vi "_getTempValueOfAllPortsTemp_EEPROM_VNA_wmg.vi"(0 "AA or AB?":bool=TRUE, 5 "portNum":i32, 7 "ref_W&R_ports":refnum<vi>[](array[refnum]), 9 "AA or AB inf":i32[](array[numeric]), 11 "info_write":string[][](array[string])) -> (4 "temp port0":string[][](array[string]), 6 "temp port1":string[][](array[string]), 10 "temp port2":string[][](array[string]), 14 "temp port4":string[][](array[string]), 15 "temp port3":string[][](array[string]))   [LabVIEW 2011]
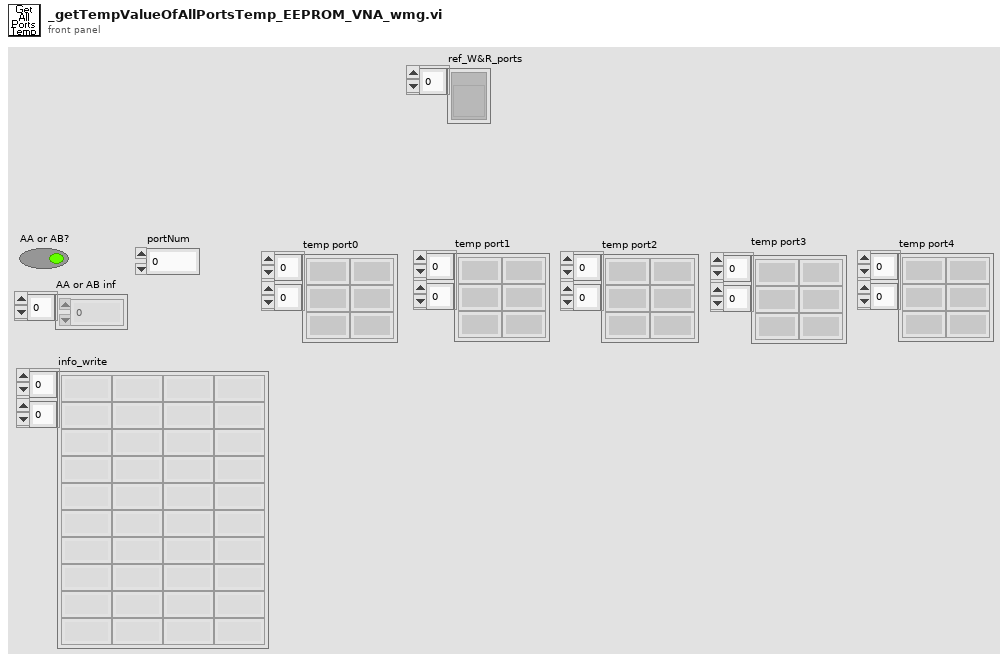
[diagram p1: front panel]
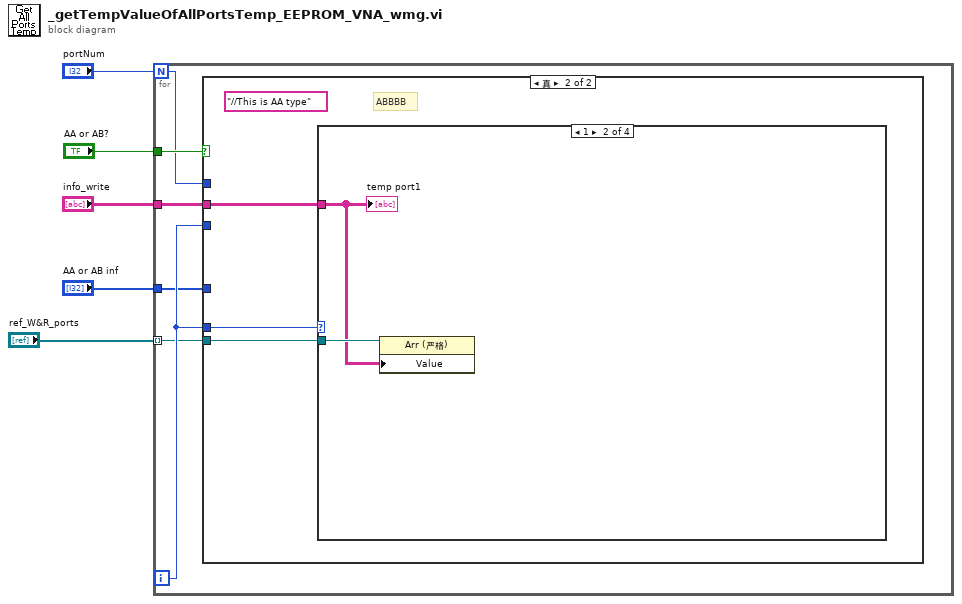
[diagram p0: block diagram]
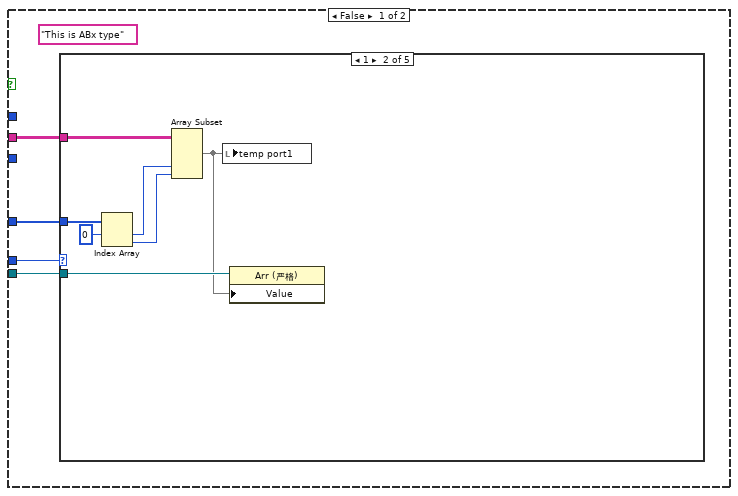
[diagram p2: hidden frame]
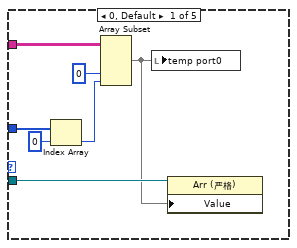
[diagram p3: hidden frame]
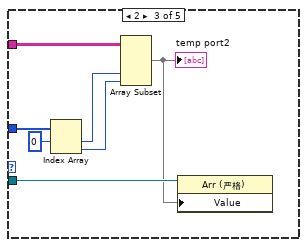
[diagram p4: hidden frame]
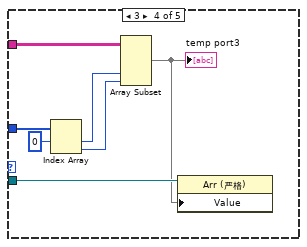
[diagram p5: hidden frame]
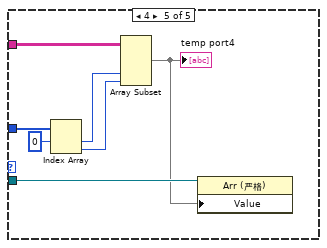
[diagram p6: hidden frame]
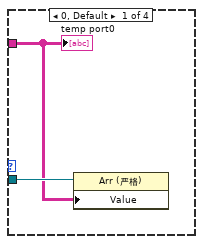
[diagram p7: hidden frame]
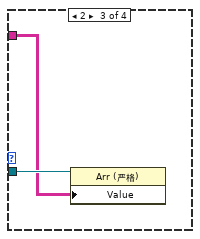
[diagram p8: hidden frame]
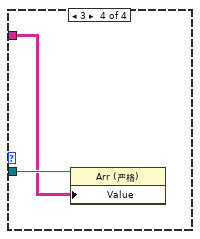
[diagram p9: hidden frame]
diagram:
  n1 = for {
    N: "portNum" -> [w8]
    tunnel: "AA or AB?" -> [w11]
    tunnel: "info_write" -> [w10]
    tunnel: "AA or AB inf" -> [w7]
    tunnel: "ref_W&R_ports" -> [w6] mode=indexing
    i -> [w9]
    n2 = case shown="真" w11 {
      tunnel: w10 -> [w14 w52]
      tunnel: w9 -> [_ _]
      tunnel: w9 -> [w15 w53]
      tunnel: w8 -> [_ _]
      tunnel: w7 -> [w13 _]
      tunnel: w6 -> [w12 w51]
      frame False {
        (unwired) "This is ABx type"
        n3 = case shown="1" w15 {
          tunnel: w14 -> [w20 w27 w34 w41 w48]
          tunnel: w13 -> [w22 w29 w36 w43 w50]
          tunnel: w12 -> [w17 w24 w31 w38 w45]
          frame 0, Default {
            n4 = Index Array(array=w22, index=0 ("索引")) -> (element=w18:i32)
            n5 = Array Subset(array=w20, index (col)=0 ("索引"), length (col)=w18) -> (w16:string[][])  [unwired: 2 in]
            n6 = local write "temp port0"(w16) -> ()
            n7 = property class="Arr (严格)"(reference=w17, "Value"=w16) -> ()  [unwired: 1 in, 2 out]
          }
          frame 1 {
            n8 = Index Array(array=w29, index #1=0 ("索引")) -> (element #1=w26:i32, element #2=w25:i32)  [unwired: 1 in]
            n9 = Array Subset(array=w27, index (col)=w26, length (col)=w25) -> (w23:string[][])  [unwired: 2 in]
            n10 = local write "temp port1"(w23) -> ()
            n11 = property class="Arr (严格)"(reference=w24, "Value"=w23) -> ()  [unwired: 1 in, 2 out]
          }
          frame 2 {
            n12 = Index Array(array=w36, index #1=0 ("索引")) -> (element #1=w33:i32, element #2=w32:i32)  [unwired: 1 in]
            n13 = Array Subset(array=w34, index (col)=w33, length (col)=w32) -> (w30:string[][])  [unwired: 2 in]
            "temp port2" <- w30
            n14 = property class="Arr (严格)"(reference=w31, "Value"=w30) -> ()  [unwired: 1 in, 2 out]
          }
          frame 3 {
            n15 = Index Array(array=w43, index #1=0 ("索引")) -> (element #1=w40:i32, element #2=w39:i32)  [unwired: 1 in]
            n16 = Array Subset(array=w41, index (col)=w40, length (col)=w39) -> (w37:string[][])  [unwired: 2 in]
            "temp port3" <- w37
            n17 = property class="Arr (严格)"(reference=w38, "Value"=w37) -> ()  [unwired: 1 in, 2 out]
          }
          frame 4 {
            n18 = Index Array(array=w50, index #1=0 ("索引")) -> (element #1=w47:i32, element #2=w46:i32)  [unwired: 1 in]
            n19 = Array Subset(array=w48, index (col)=w47, length (col)=w46) -> (w44:string[][])  [unwired: 2 in]
            "temp port4" <- w44
            n20 = property class="Arr (严格)"(reference=w45, "Value"=w44) -> ()  [unwired: 1 in, 2 out]
          }
        }
      }
      frame True {
        (unwired) "//This is AA type"
        # "ABBBB"
        n21 = case shown="1" w53 {
          tunnel: w52 -> [w54 w56 w58 w60]
          tunnel: w51 -> [w55 w57 w59 w61]
          frame 0, Default {
            n22 = property class="Arr (严格)"(reference=w55, "Value"=w54) -> ()  [unwired: 1 in, 2 out]
            "temp port0" <- w54
          }
          frame 1 {
            n23 = property class="Arr (严格)"(reference=w57, "Value"=w56) -> ()  [unwired: 1 in, 2 out]
            "temp port1" <- w56
          }
          frame 2 {
            n24 = property class="Arr (严格)"(reference=w59, "Value"=w58) -> ()  [unwired: 1 in, 2 out]
          }
          frame 3 {
            n25 = property class="Arr (严格)"(reference=w61, "Value"=w60) -> ()  [unwired: 1 in, 2 out]
          }
        }
      }
    }
  }
